vi "TCP-Combine Address and Port.vi"(5 "Address":string, 9 "Port":i32) -> (8 "Address out":string)   [LabVIEW 2020]
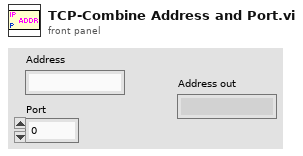
[diagram p1: front panel]
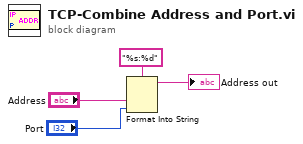
[diagram p0: block diagram]
diagram:
  n1 = Format Into String(format string="%s:%d", "Address", "Port") -> (resulting string=→"Address out":string)  [unwired: 2 in, 1 out]
